vi "Open.vi"(8 "error in":errorcluster, 9 "parameters":variant, 10 "file path":path, 11 "SystemConfigRepo in":refnum<class "SystemConfigRepo.lvclass">) -> (0 "error out":errorcluster, 2 "invalid?":bool, 3 "SystemConfigRepo out":refnum<class "SystemConfigRepo.lvclass">)   [LabVIEW 2013, in "PL Framework Configuration Tool.lvlib" / "SystemConfigRepo.lvclass"]
uses:
  SystemConfigRepo.lvclass
  SystemConfigRepo.lvclass/SystemConfigRepo.ctl
  Framework Configuration Classes/platypus configuration/PLConfigurationSerializer.lvlib
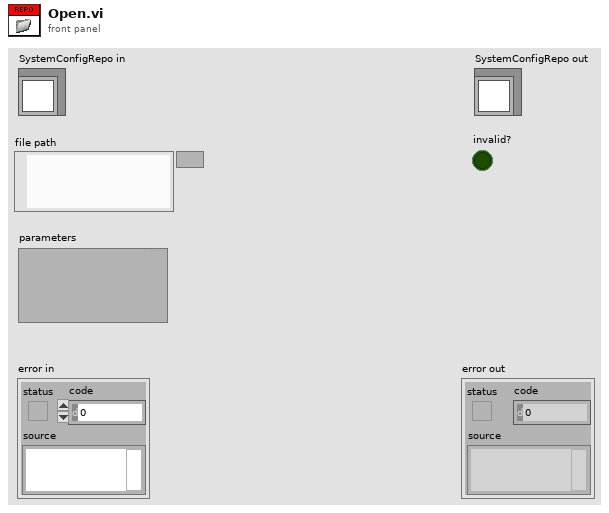
[diagram p1: front panel]
types:
  T1 = typedef "PLConfigurationSerializer.lvlib/systems cluster.ctl" = cluster{"System Configuration":refnum<class "PL_System Configuration.lvclass">, "targets":T2[]}
  T2 = typedef "PLConfigurationSerializer.lvlib/targets cluster.ctl" = cluster{"Target Configuration":refnum<class "PL_Target Configuration.lvclass">, "engines":T3[]}
  T3 = typedef "PLConfigurationSerializer.lvlib/engines cluster.ctl" = cluster{"engine configuration":refnum<class "engine configuration.lvclass">, "modules":refnum<class "TBM module configuration.lvclass">[]}
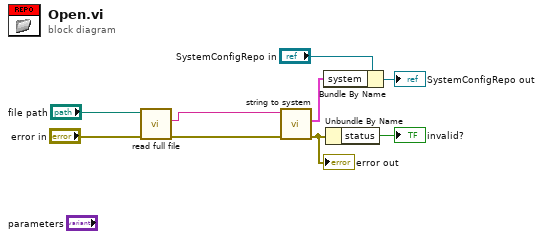
[diagram p0: block diagram]
diagram:
  n1 = call "read full file.vi"("error in"="error in", "file path"="file path") -> ("error out"=w1:errorcluster, "data"=w6:string)  [unwired: 8 in]
  n2 = call "string to system.vi"("error in"=w1, "data"=w6) -> ("error out"=w5:errorcluster, "system"=w2:T1)  [unwired: 8 in]
  "error out" <- w5
  n3 = Bundle By Name(cluster="SystemConfigRepo in", "system"=w2) -> (→"SystemConfigRepo out":refnum<class "SystemConfigRepo.lvclass">)
  n4 = Unbundle By Name(w5) -> ("status"=→"invalid?":bool)
